vi "Generic command handler.vi"(8 "error in (no error)":errorcluster, 10 "Message in":refnum<class "GenericMessage.lvclass">, 11 "Murmex in":refnum<class "ExampleClassA.lvclass">) -> (0 "error out":errorcluster, 2 "value":string, 3 "Murmex out":refnum<class "ExampleClassA.lvclass">)   [LabVIEW 2012, in "ExampleClassA.lvclass"]
doc: "Handles the generic command \"proceed\" (only used internally) to repeatedly produce/stream data."
uses:
  ExampleClassA.lvclass
  <vilib>/Distrio/Murmex/GenericMessage/GenericMessage.lvclass
  <vilib>/Distrio/Murmex/Murmex/Murmex.lvclass
  ExampleClassA.lvclass/ExampleClassA.ctl
  <vilib>/Distrio/Murmex/StopMessage/StopMessage.lvclass
  <vilib>/Distrio/Murmex/Message/Add or replace parameter.vi
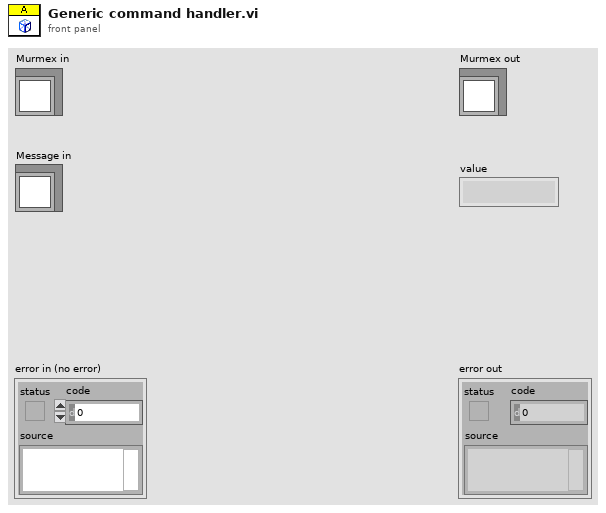
[diagram p1: front panel]
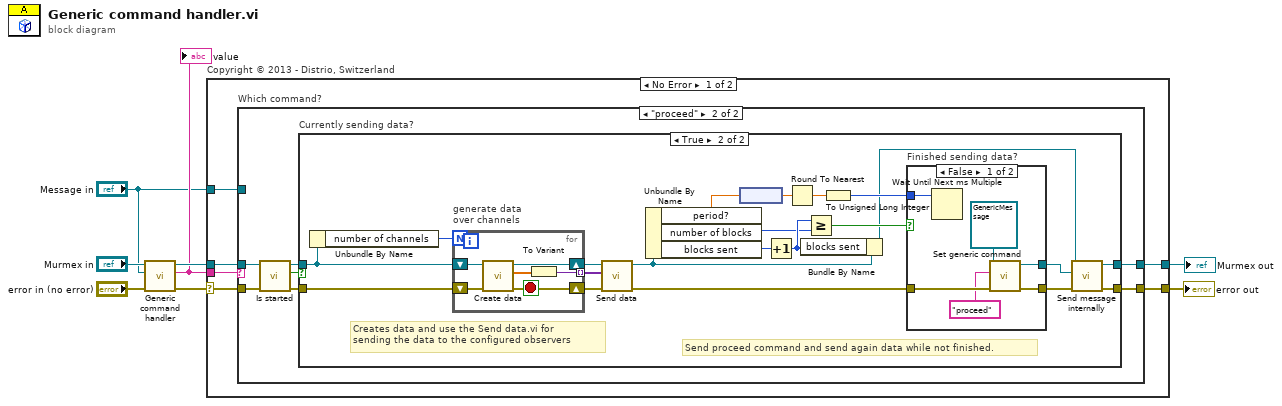
[diagram p0: block diagram]
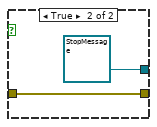
[diagram p4: hidden frame]
diagram:
  n1 = call-parent "Generic command handler.vi"("error in (no error)"="error in (no error)", "Message in"="Message in", "Murmex in"="Murmex in") -> ("error out"=w8:errorcluster, "value"=w2:string, "Murmex out"=w7:refnum<class "ExampleClassA.lvclass">)  [unwired: 6 in]
  "value" <- w2
  n2 = case "Copyright © 2013 - Distrio, Switzerland" shown="No Error" w8 {
    selector: w8 -> [w13 w62]
    tunnel: w7 -> [w12 w61]
    tunnel: [w11 w62] -> w4
    tunnel: w2 -> [w14 _]
    tunnel: [w10 w61] -> w3
    tunnel: "Message in" -> [w9 _]
    frame No Error {
      n3 = case "Which command?" shown="\"proceed\"" w14 {
        tunnel: w13 -> [w15 w23]
        tunnel: [w16 w17] -> w10
        tunnel: w12 -> [w16 w22]
        tunnel: [w15 w18] -> w11
        tunnel: w9 -> [_ _]
        frame Default {
        }
        frame "proceed" {
          n4 = call <vilib>:"Is started.vi"("error in (no error)"=w23, "Murmex in"=w22) -> ("error out"=w21:errorcluster, "started?"=w19:bool, "Murmex out"=w20:refnum<class "ExampleClassA.lvclass">)  [unwired: 7 in]
          n5 = case "Currently sending data?" shown="True" w19 {
            tunnel: w21 -> [w24 w29]
            tunnel: w20 -> [w25 w32]
            tunnel: [w24 w35] -> w18
            tunnel: [w25 w36] -> w17
            frame False {
            }
            frame True {
              # "Send proceed command and send again data while not finished."
              # "Creates data and use the Send data.vi for\nsending the data to the configured observers"
              n6 = Unbundle By Name(w32) -> ("number of channels"=w31:i32)
              n7 = for "generate data\nover channels" {
                N: w31 -> [_]
                shift-right: [w52] -> w46
                shift-left: w32 -> [w50]
                shift-right: [w49] -> w28
                shift-left: w29 -> [w51]
                tunnel: [w47] -> w30 mode=indexing
                stop <- w49 stop-if-true
                n8 = call "Create data.vi"("error in (no error)"=w51, "Example Class A in"=w50) -> ("error out"=w49:errorcluster, "Graph"=w48:dbl[], "Example Class A out"=w52:refnum<class "ExampleClassA.lvclass">)  [unwired: 7 in]
                n9 = To Variant(anything=w48) -> (Variant=w47:variant)
              }
              n10 = call <vilib>:"Send data.vi"("error in (no error)"=w28, "data (channels array)"=w30, "Murmex in"=w46) -> ("error out"=w27:errorcluster, "Murmex out"=w41:refnum<class "ExampleClassA.lvclass">)  [unwired: 7 in]
              n11 = Unbundle By Name(w41) -> ("period?"=w45:dbl[unit], "number of blocks"=w38:i32, "blocks sent"=w40:i32)
              n12 = node(w45) -> (w44:dbl)
              n13 = Increment(x=w40) -> (x+1=w39:i32)
              n14 = Round To Nearest(number=w44) -> (nearest integer value=w43:dbl)
              n15 = Bundle By Name(cluster=w41, "blocks sent"=w39) -> (w34:refnum<class "ExampleClassA.lvclass">)
              n16 = Greater Or Equal?(x=w39, y=w38) -> (x >= y?=w37:bool)
              n17 = To Unsigned Long Integer(number=w43) -> (unsigned 32bit integer=w42:u32)
              n18 = case "Finished sending data?" shown="False" w37 {
                tunnel: w27 -> [w57 w60]
                tunnel: w42 -> [w58 _]
                tunnel: [w54 w60] -> w26
                tunnel: [w55 refnum<class "StopMessage.lvclass"> refnum ("StopMessage.lvclass")] -> w33
                frame False {
                  n19 = Wait Until Next ms Multiple(millisecond multiple=w58) -> ()  [unwired: 1 out]
                  n20 = call <vilib>:"Set generic command.vi"("error in (no error)"=w57, "generic command"="proceed" ("command string"), "GenericMessage in"=refnum<class "GenericMessage.lvclass"> refnum ("GenericMessage.lvclass")) -> ("error out"=w54:errorcluster, "GenericMessage out"=w55:refnum<class "GenericMessage.lvclass">)  [unwired: 7 in]
                }
                frame True {
                }
              }
              n21 = call <vilib>:"Send message internally.vi"("error in (no error)"=w26, "Message"=w33, "Murmex in"=w34) -> ("error out"=w35:errorcluster, "Murmex out"=w36:refnum<class "ExampleClassA.lvclass">)  [unwired: 7 in]
            }
          }
        }
      }
    }
    frame Error {
    }
  }
  "error out" <- w4
  "Murmex out" <- w3
